vi "Valco Valve Mngr.vi"(0 "Valve":T1=enum."Well 2", 1 "Mngr Action":T3, 5 "Cmd":string, 9 "Valve Config":T2, 11 "error in (no error)":errorcluster) -> (6 "Com Log":string, 8 "Output Value":dbl caption="Current Position(half steps)", 13 "Move Successful":bool, 14 "Connected":bool, 15 "error out":errorcluster)   [LabVIEW 2018]
uses:
  Valco Valve/Valco Valve Mngr Action.ctl
  Valco Valve/Valco Valve Config.ctl
  Main/Drain Valve.ctl
  Lib/Serial/Find Device Protocols.ctl
  Hardware Globals.vi
  Lib/Utilities.lvlib
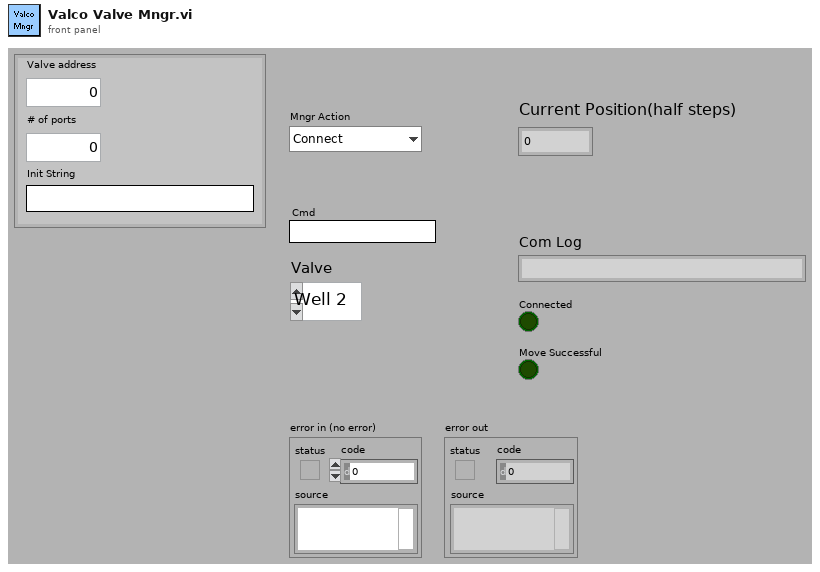
[diagram p1: front panel]
types:
  T1 = typedef "Drain Valve.ctl" = enum16{"Well 1", "Well 2", "Well 3", "Well 4", "Well X"}
  T2 = typedef "Valco Valve Config.ctl" = cluster{"Valve address":u32, "# of ports":u32, "Init String":string}
  T3 = typedef "Valco Valve Mngr Action.ctl" = enum16{"Connect", "Init", "Cmd", "Set Valve", "Status", "Close"}
  T4 = typedef "Find Device Protocols.ctl" = enum16{"Init", "RS232(no baud)", "RS232", "RS485", "USB", "GPIB", "Ethernet"}
  T5 = enum16{"Init", "Reset", "Read", "Update", "Close"}
  T6 = cluster{"negative limit switch":bool, "positive limit switch":bool, "home switch":bool, "position marker":bool, "device enable":bool, "quick stop":bool, "general purpose J":bool, "general purpose I":bool, "general purpose H":bool, "general purpose G":bool, "general purpose F":bool, "general purpose E":bool, "general purpose D":bool, "general purpose C":bool, "general purpose B":bool, "general purpose A":bool}
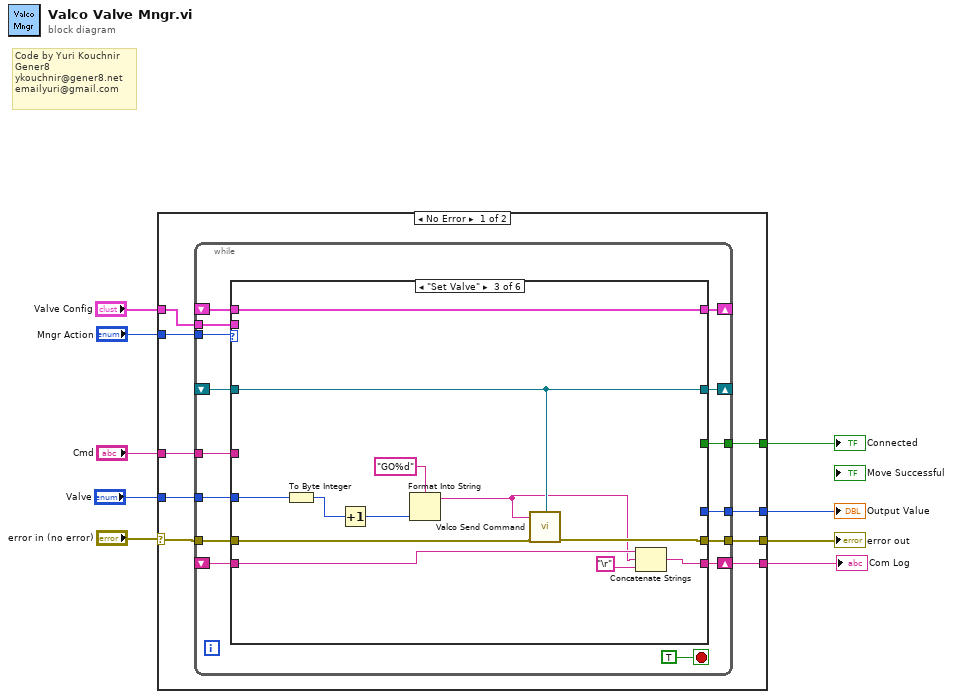
[diagram p0: block diagram]
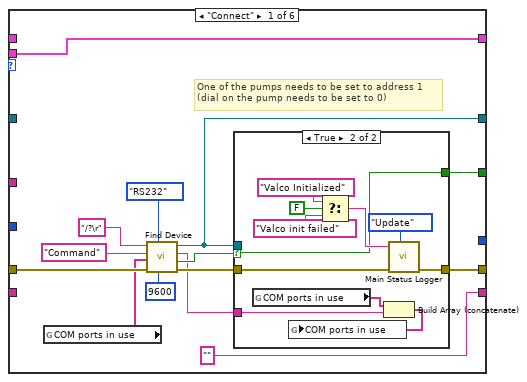
[diagram p2: hidden frame]
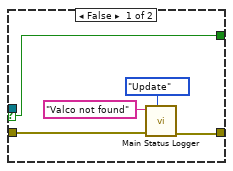
[diagram p3: hidden frame]
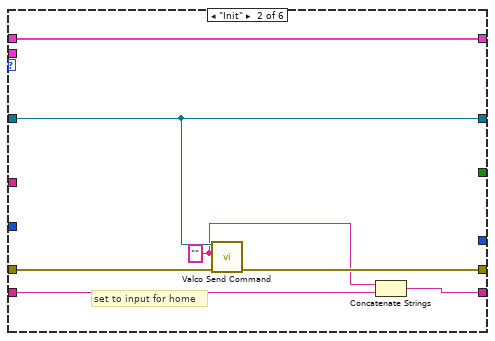
[diagram p4: hidden frame]
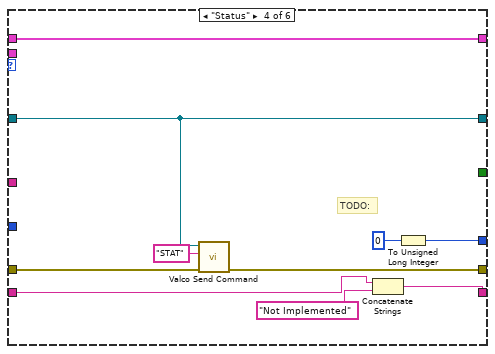
[diagram p5: hidden frame]
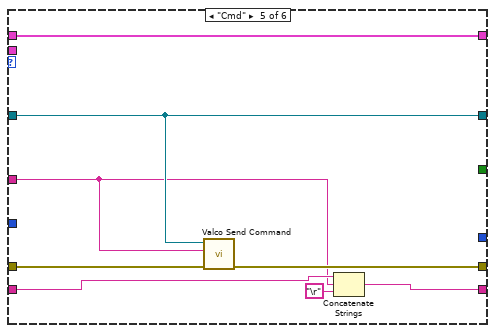
[diagram p6: hidden frame]
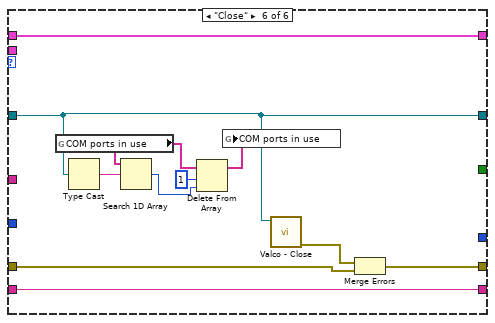
[diagram p7: hidden frame]
diagram:
  # "Code by Yuri Kouchnir\nGener8\nykouchnir@gener8.net\nemailyuri@gmail.com"
  n1 = case shown="No Error" "error in (no error)" {
    selector: "error in (no error)" -> [w18 w112]
    tunnel: [w17 w112] -> w8
    tunnel: "Mngr Action" -> [w16 _]
    tunnel: [w15 _] -> w6
    tunnel: [w14 _] -> w5
    tunnel: "Cmd" -> [w13 _]
    tunnel: [w12 _] -> w3
    tunnel: "Valve Config" -> [w11 _]
    tunnel: "Valve" -> [w10 _]
    frame No Error {
      n2 = while {
        tunnel: w18 -> [w31]
        tunnel: [w30] -> w17
        tunnel: w16 -> [w32]
        tunnel: [w29] -> w15
        shift-right: [w28] -> _
        shift-left: _ -> [w27]
        tunnel: [w26] -> w14
        tunnel: w13 -> [w25]
        shift-right: [w23] -> _
        shift-left: _ -> [w21]
        tunnel: w11 -> [w22]
        shift-right: [w24] -> w12
        shift-left: _ -> [w20]
        tunnel: w10 -> [w19]
        stop <- TRUE stop-if-true
        n3 = case shown="\"Set Valve\"" w32 {
          tunnel: w31 -> [w46 w67 w82 w92 w100 w111]
          tunnel: [w47 w69 w81 w91 w99 w110] -> w30
          tunnel: [w42 _ _ _ _ _] -> w29
          tunnel: [w41 w70 w80 w90 w98 w107] -> w28
          tunnel: w27 -> [_ w70 w80 w90 w98 w107]
          tunnel: [_ _ _ w87 _ _] -> w26
          tunnel: w25 -> [_ _ _ _ w94 _]
          tunnel: ["" ("ID Response") w65 w78 w86 w97 w101] -> w24
          tunnel: [w35 w68 w79 w88 w96 w108] -> w23
          tunnel: w22 -> [w35 _ _ _ _ _]
          tunnel: w21 -> [_ w68 w79 w88 w96 w108]
          tunnel: w20 -> [_ w66 w77 w85 w95 w101]
          tunnel: w19 -> [_ _ w73 _ _ _]
          frame "Connect" {
            # "One of the pumps needs to be set to address 1\n(dial on the pump needs to be set to 0)"
            n4 = global read "Hardware Globals.vi" "COM ports in use"() -> (w37:string[])
            n5 = call "Find Device.vi"("Baud Rate"=u32 9600, "Device Type"=Find_Device_Protocols."RS232", "error in (no error)"=w46, "Ports in Use"=w37, "ID Response"="Command", "ID String"="/?\r") -> ("error out"=w45:errorcluster, "Device Found"=w43:bool, "device ID"=w38:string, "VISA resource name out"=w41:refnum<visa-resource-name>)  [unwired: 1 in, 1 out]
            n6 = case shown="True" w43 {
              selector: w43 -> [w52 w54]
              tunnel: [w49 w59] -> w47
              tunnel: w45 -> [w50 w55]
              tunnel: [w52 w54] -> w42
              tunnel: w41 -> [_ _]
              tunnel: w38 -> [_ w56]
              frame False {
                n7 = call "Main Status Logger.vi"("Action"=T5."Update", "error in"=w50, "Input String"="Valco not found") -> ("error out"=w49:errorcluster)  [unwired: 7 in, 1 out]
              }
              frame True {
                n8 = global read "Hardware Globals.vi" "COM ports in use"() -> (w58:string[])
                n9 = Select(t="Valco Initialized" ("ID Response"), s=FALSE, f="Valco init failed" ("ID Response")) -> (s? t:f=w60:string)
                n10 = Build Array (concatenate)(w58, w56) -> (w57:string[])
                n11 = global write "Hardware Globals.vi" "COM ports in use"(w57) -> ()
                n12 = call "Main Status Logger.vi"("Action"=T5."Update", "error in"=w55, "Input String"=w60) -> ("error out"=w59:errorcluster)  [unwired: 7 in, 1 out]
              }
            }
          }
          frame "Init" {
            w64 = "" ("Command")
            # "set to input for home"
            n13 = call "Valco Send Command.vi"("error in (no error)"=w67, "Command"=w64, "VISA resource name in"=w70) -> ("error out"=w69:errorcluster)  [unwired: 7 in, 1 out]
            n14 = Concatenate Strings(w64, w66) -> (w65:string)
          }
          frame "Set Valve" {
            n15 = To Byte Integer(number=w73) -> (8bit integer=w72:i8)
            n16 = Increment(x=w72) -> (x+1=w71:i8)
            n17 = Format Into String(format string="GO%d", w71) -> (resulting string=w74:string)  [unwired: 2 in, 1 out]
            n18 = call "Valco Send Command.vi"("error in (no error)"=w82, "Command"=w74, "VISA resource name in"=w80) -> ("error out"=w81:errorcluster)  [unwired: 7 in, 1 out]
            n19 = Concatenate Strings(w77, w74, "\r") -> (w78:string)
          }
          frame "Status" {
            # "TODO:"
            n20 = call "Valco Send Command.vi"("error in (no error)"=w92, "Command"="STAT", "VISA resource name in"=w90) -> ("error out"=w91:errorcluster)  [unwired: 7 in, 1 out]
            n21 = Concatenate Strings(w85, "Not Implemented" ("string")) -> (w86:string)
            n22 = To Unsigned Long Integer(number=u32 0) -> (unsigned 32bit integer=w87:u32)
          }
          frame "Cmd" {
            n23 = call "Valco Send Command.vi"("error in (no error)"=w100, "Command"=w94, "VISA resource name in"=w98) -> ("error out"=w99:errorcluster)  [unwired: 7 in, 1 out]
            n24 = Concatenate Strings(w95, w94, "\r") -> (w97:string)
          }
          frame "Close" {
            n25 = global read "Hardware Globals.vi" "COM ports in use"() -> (w105:string[])
            n26 = Type Cast(x=w107) -> (*(type *) &x=w106:string)  [unwired: 1 in]
            n27 = Search 1D Array(1D array=w105, element=w106) -> (index of element=w103:i32)  [unwired: 1 in]
            n28 = Delete From Array(array=w105, length=1, index=w103) -> (array with subset deleted=w102:string[])  [unwired: 1 out]
            n29 = global write "Hardware Globals.vi" "COM ports in use"(w102) -> ()
            n30 = call "Valco - Close.vi"("VISA resource name"=w107) -> ("error out"=w109:errorcluster)  [unwired: 10 in]
            n31 = Merge Errors(w109, w111) -> (w110:errorcluster)
          }
        }
      }
    }
    frame Error {
      (unwired) T6 {"negative limit switch"=FALSE, "positive limit switch"=FALSE, "home switch"=FALSE, "position marker"=FALSE, "device enable"=FALSE, "quick stop"=FALSE, "general purpose J"=FALSE, "general purpose I"=FALSE, "general purpose H"=FALSE, "general purpose G"=FALSE, "general purpose F"=FALSE, "general purpose E"=FALSE, "general purpose D"=FALSE, "general purpose C"=FALSE, "general purpose B"=FALSE, "general purpose A"=FALSE} ("digital inputs")
    }
  }
  "error out" <- w8
  "Connected" <- w6
  "Output Value" <- w5
  "Com Log" <- w3
